vi "sub_force_buf.vi"(7 "cmd":T1, 8 "error in":errorcluster, 11 "forcewf":waveform(dbl) caption="Waveform") -> (0 "error out":errorcluster, 3 "queue out":refnum<queue>)   [LabVIEW 2016]
uses:
  ctl/Data_buf_cmd.ctl
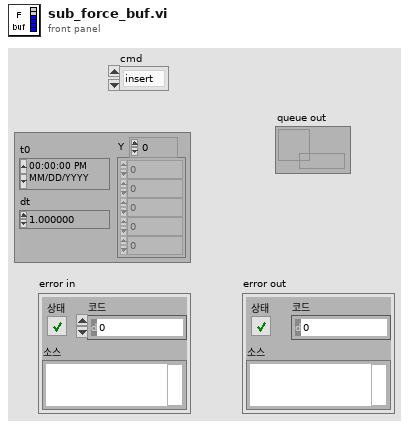
[diagram p1: front panel]
types:
  T1 = typedef "Data_buf_cmd.ctl" = enum16{"insert", "default", "create", "clear"}
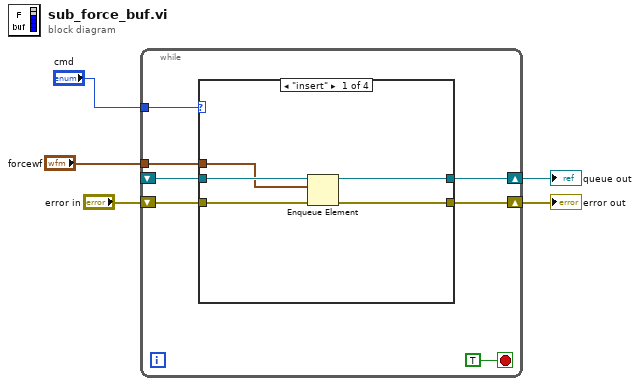
[diagram p0: block diagram]
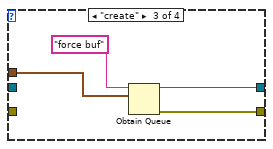
[diagram p3: hidden frame]
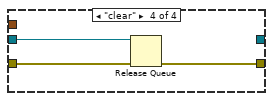
[diagram p4: hidden frame]
diagram:
  n1 = while {
    shift-right: [w9] -> w1
    shift-left: _ -> [w10]
    tunnel: "cmd" -> [w11]
    shift-right: [w7] -> w4
    shift-left: "error in" -> [w8]
    tunnel: "forcewf" -> [w6]
    stop <- TRUE stop-if-true
    n2 = case shown="\"insert\"" w11 {
      tunnel: w10 -> [w17 w19 _ w26]
      tunnel: [w16 w19 w23 _] -> w9
      tunnel: w8 -> [w15 w18 _ w25]
      tunnel: [w14 w18 w22 w24] -> w7
      tunnel: w6 -> [w13 _ w21 _]
      frame "insert" {
        n3 = Enqueue Element(queue=w17, element=w13, error in (no error)=w15) -> (queue out=w16:refnum<queue>, error out=w14:errorcluster)  [unwired: 1 in, 1 out]
      }
      frame "default", Default {
      }
      frame "create" {
        n4 = Obtain Queue(name (unnamed)="force buf" ("이름(이름없음)"), element data type=w21) -> (queue out=w23:refnum<queue>, error out=w22:errorcluster)  [unwired: 3 in, 1 out]
      }
      frame "clear" {
        n5 = Release Queue(queue=w26, error in (no error)=w25) -> (error out=w24:errorcluster)  [unwired: 1 in, 2 out]
      }
    }
  }
  "error out" <- w4
  "queue out" <- w1
